vi "Monitor.vi"() -> ()   [LabVIEW 2017]
uses:
  Run_vi2.xctl
  <vilib>/Utility/miscctls.llb/LVPointTypeDef.ctl
  Global_comSerie.vi
  <vilib>/Instr/_visa.llb/VISA Configure Serial Port (Instr).vi
  GlobalFag.vi
  <vilib>/addons/database/Connection.llb/DB Tools Open Connec (Path).vi
  Global_linker_path_logger.vi
  contador_logger_global.vi
  global_act_eje_aula.vi
  global_act_eje_edif.vi
  Global_linker_path_3.vi
  <vilib>/addons/database/_DB Variant To Data/Database Variant To Data.xnode
  <vilib>/addons/database/NI_Database_API.lvlib
panel:
  in  "Periodo (s)":dbl=20.0 caption="Time Target (s)"
  out "Numeric":i32
  in  "Run_vi2":dbl(xcontrol)
  out "+/-_2":bool
  out "bit_edo_+/-_2":bool
  out "bit_edo_+/-":bool
  out "+/-":bool
  out "A_fin":u8
  out "A_ini":u8
  out "rango_TRUE":bool
  out "range":u8
  out "servicio_hex 2":string
  out "Edificio_ 2":string
  out "Hora_Inicio as string 2":string
  out "Hora_Inicio_as Time stamp 2":timestamp format="%<%X>T"
  out "Tarea Aula_ok":bool
  out "Aula":string
  out "ID a ejecutar":string
  out "hora_hoy as string 2":string
  out "Table Control_aulas":string[][](table) caption="Tarea por Aula"
  out "size_aulas":i32[](array[numeric])
  in  "Programar Tareas2":bool
  in  "Home Button":bool
  out "ID a ejecutar":string
  out "servicio_hex":string
  out "Edificio_":string
  out "Hora_Inicio as string":string
  out "Hora_Inicio_as Time stamp 1":timestamp format="%<%X>T"
  out "tarea_edif_ok":bool
  out "hora_hoy as string":string
  out "Table Control":string[][](table) caption="Tareas por Edificio"
  out "size(s)":i32[](array[numeric])
  in  "Ejecutor de Tareas":bool
  in  "Programar Tareas":bool
  out "inc_1":bool
  out "inc_2":bool
  out "inc_3":bool
  out "inc_4":bool
  out "inc_5":bool
  out "inc_6":bool
  out "inc_7":bool
  out "inc_8":bool
  out "inc_9":bool
  out "inc_10":bool
  out "inc_11":bool
  out "inc_12":bool
  out "inc_16":bool
  out "inc_15":bool
  out "inc_14":bool
  out "inc_13":bool
  in  "Puerto Serial":refnum<visa-resource-name>="COM1"
  out "A_16":bool[](array[boolean])
  out "A_15":bool[](array[boolean])
  out "A_14":bool[](array[boolean])
  out "A_13":bool[](array[boolean])
  out "A_12":bool[](array[boolean])
  out "A_11":bool[](array[boolean])
  out "A_10":bool[](array[boolean])
  out "A_9":bool[](array[boolean])
  out "A_8":bool[](array[boolean])
  out "A_7":bool[](array[boolean])
  out "A_6":bool[](array[boolean])
  out "A_5":bool[](array[boolean])
  out "A_4":bool[](array[boolean])
  out "A_3":bool[](array[boolean])
  out "A_2":bool[](array[boolean])
  out "A_1":bool[](array[boolean])
  in  "Stop Button":bool
  in  "Manual Aula / Edificio":bool
  # "Edificio A"
  # "Ejecutor de Tareas"
  # "a"
  # "b"
  # "c"
  # "d"
  # "e"
  # "Aula"
  # "1"
  # "a.- Luz\nb.- Aire\nc.- Proyector\nd.- Agua\ne.- Acceso"
  # "2"
  # "3"
  # "4"
  # "5"
  # "Servicios:"
  # "6"
  # "a  Luz"
  # "7"
  # "b  Aire"
  # "8"
  # "c  Proyector"
  # "d  Agua"
  # "9"
  # "e  Acceso"
  # "10"
  # "11"
  # "12"
  # "13"
  # "14"
  # "15"
  # "16"
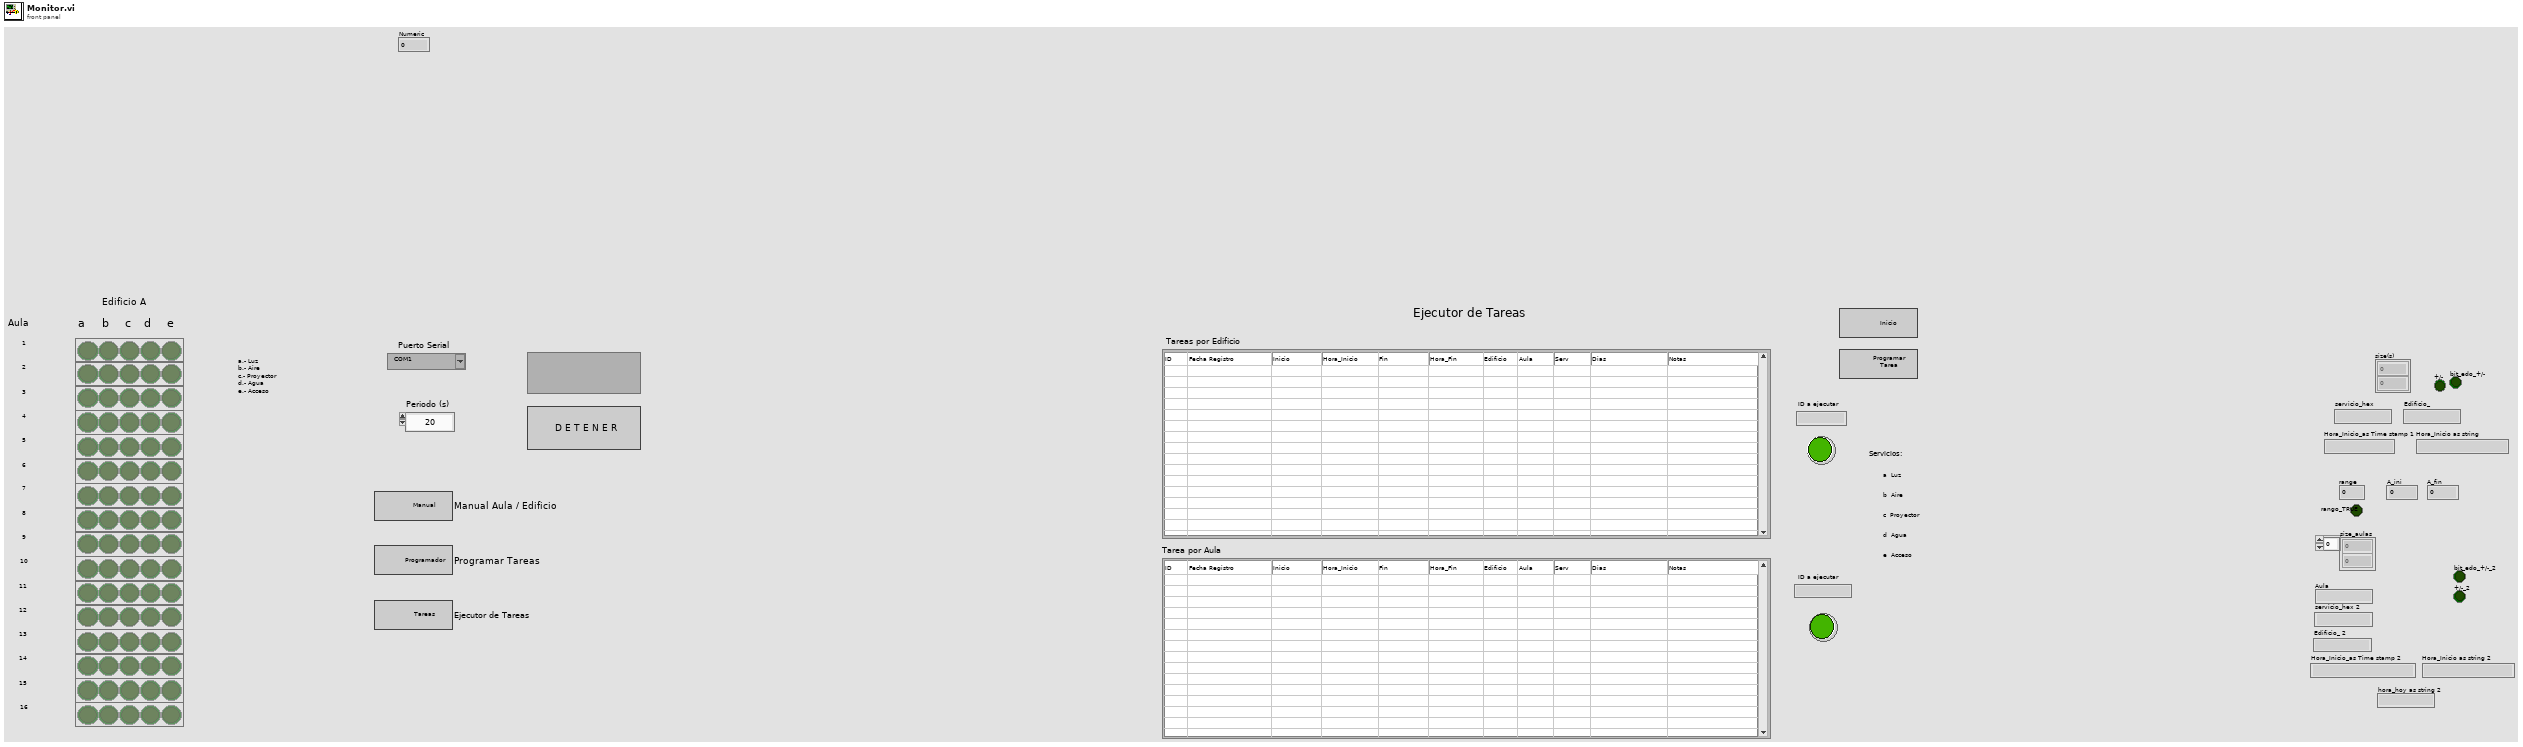
[diagram p1: front panel]
types:
  T1 = enum16{"open", "replace", "create", "open or create", "replace or create", "replace or create with confirmation"}
  T2 = typedef "LVPointTypeDef.ctl" = cluster{"Horizontal":i16, "Vertical":i16}
  T3 = typedef "NI_Database_API.lvlib/Conn ObjectReference.ctl" = refnum<k1>
  T4 = cluster{u64, string, "read buffer":string, u8, "serv":string}
  T5 = enum32{"Invalid", "Standard", "Closed", "Hidden", "Minimized", "Maximized"}
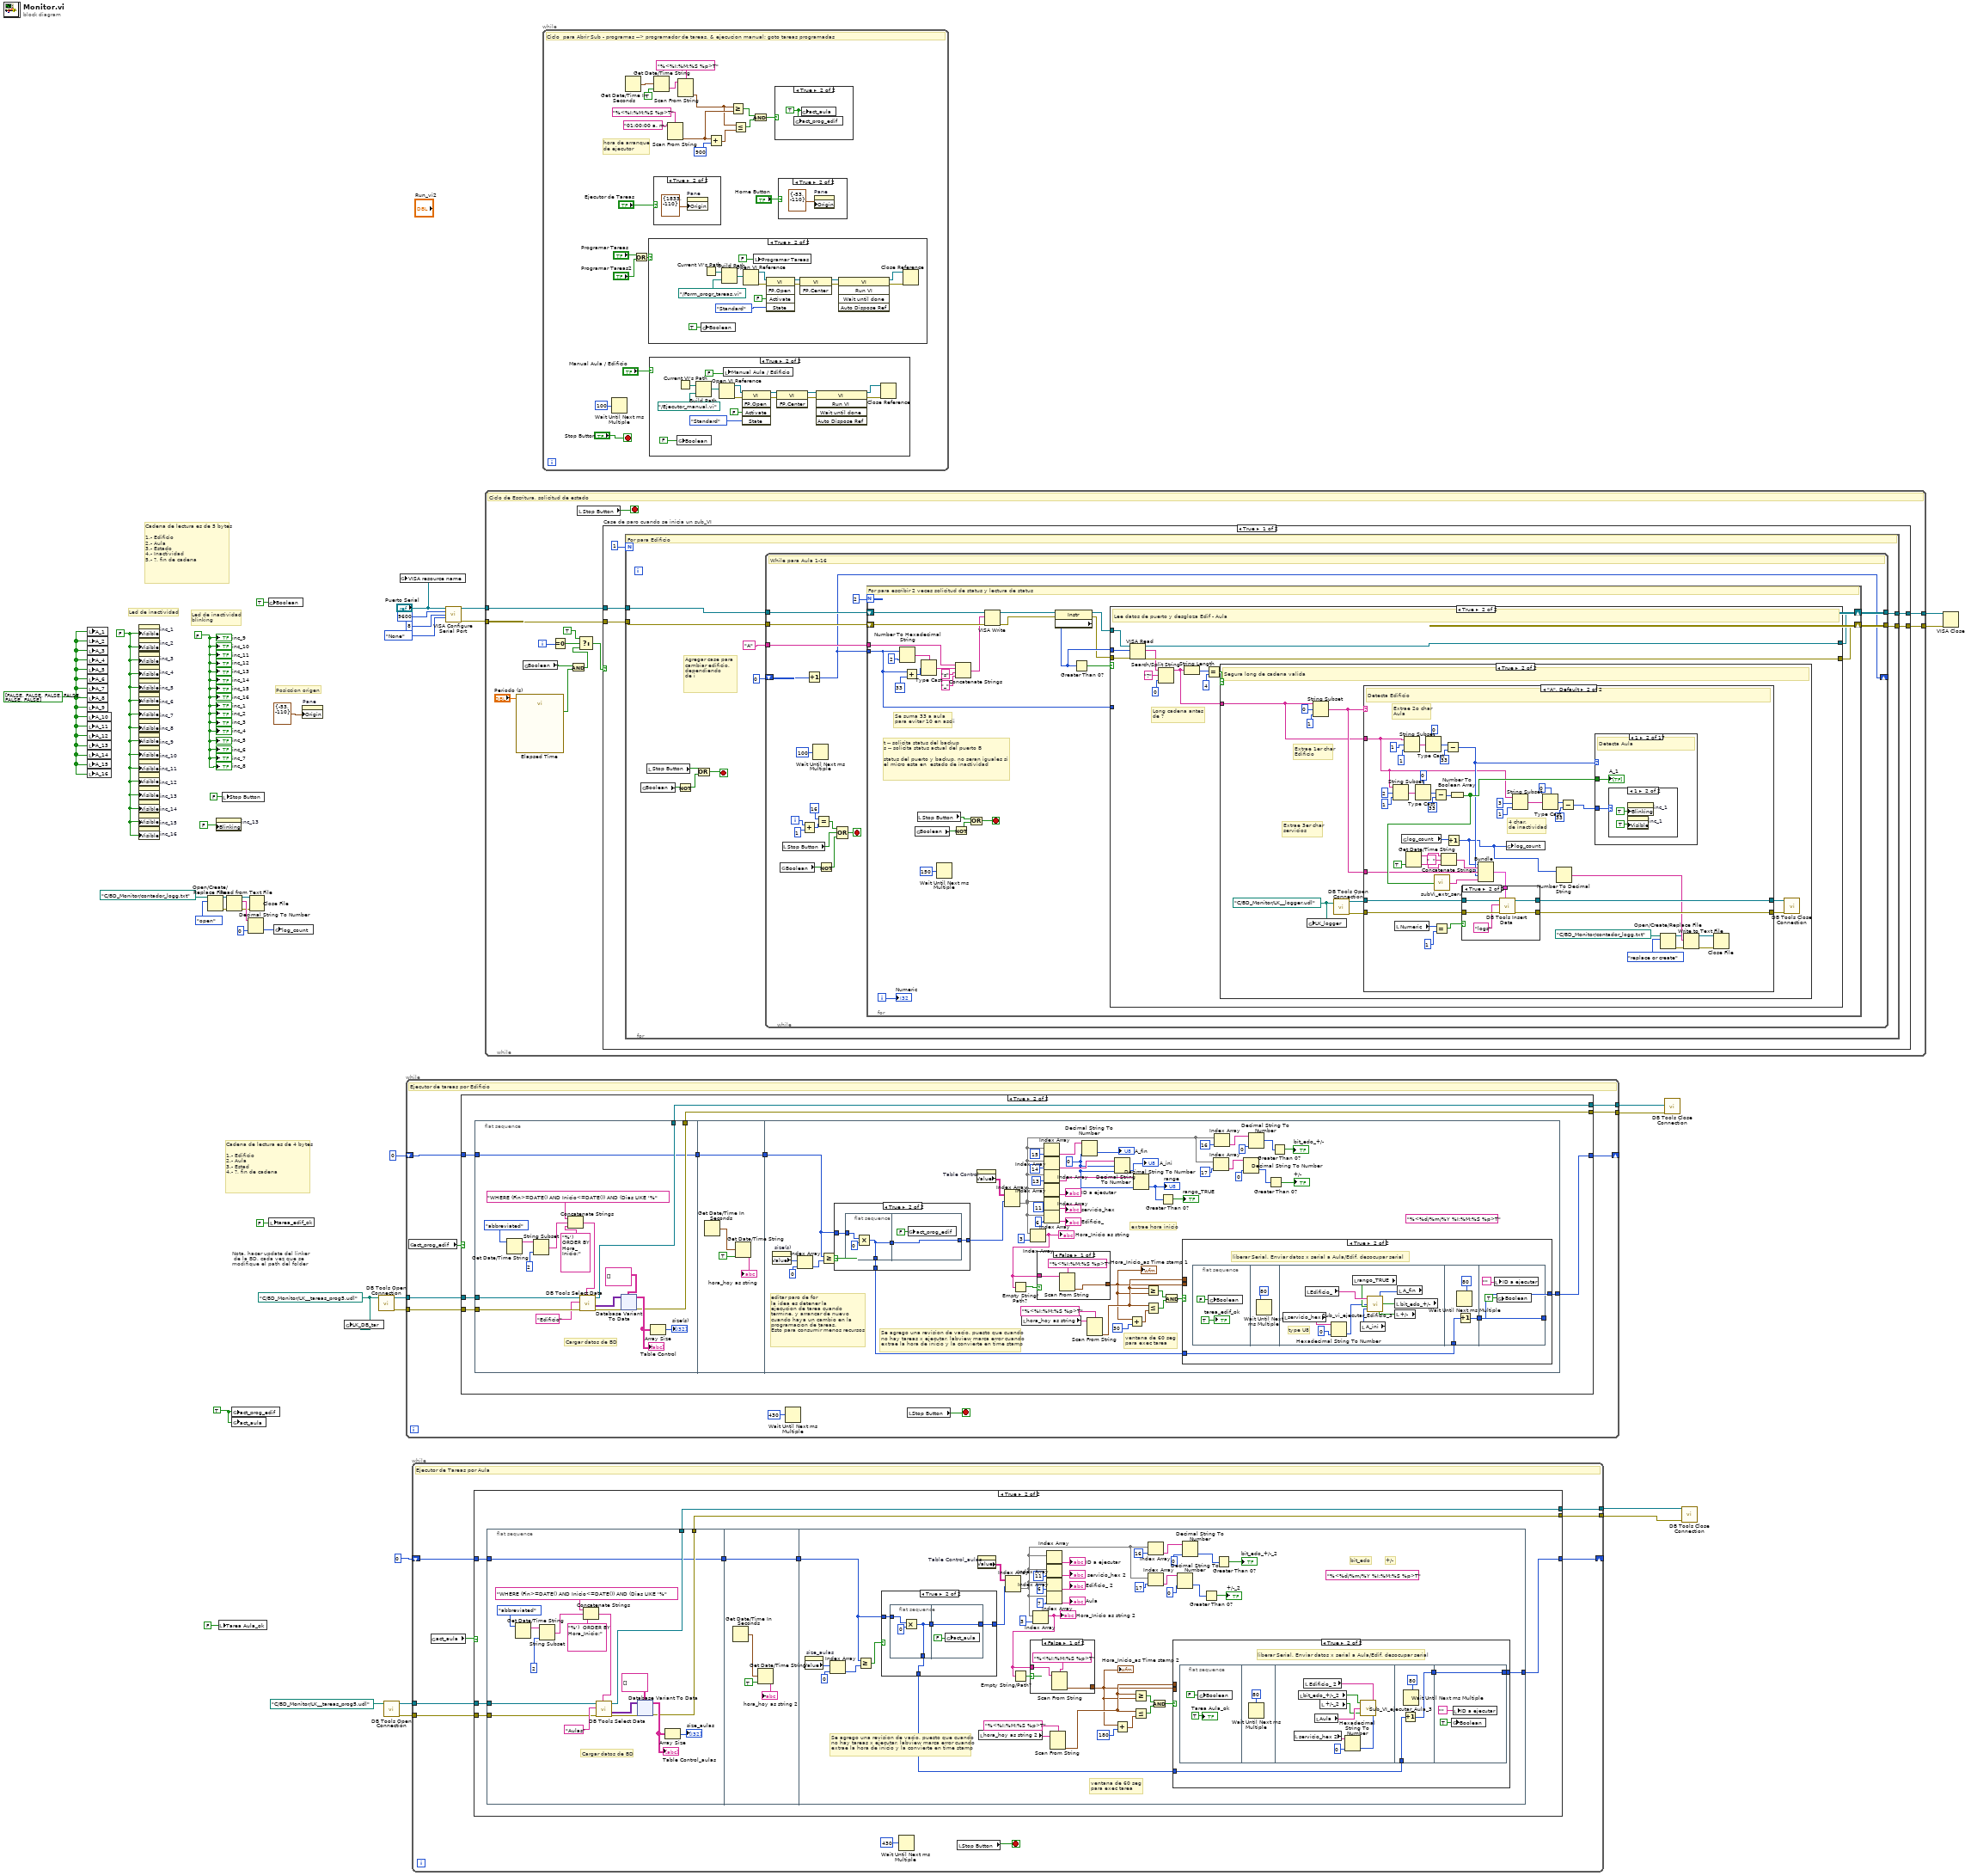
[diagram p0: block diagram]
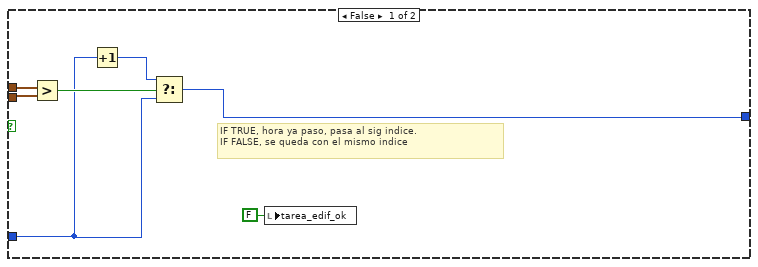
[diagram p4: hidden frame]
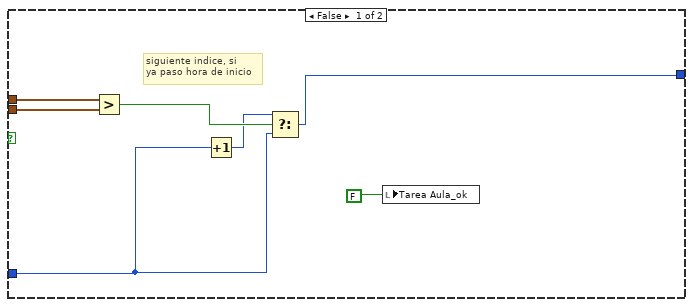
[diagram p8: hidden frame]
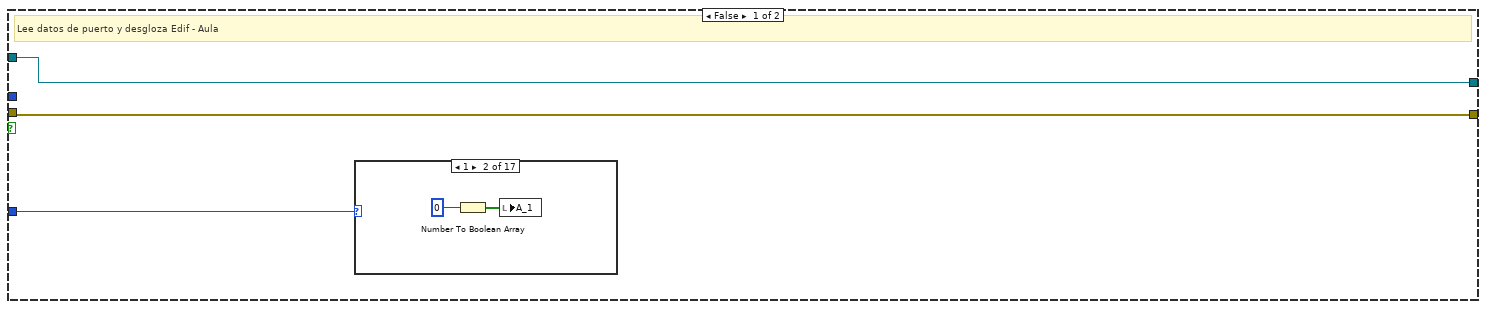
[diagram p15: hidden frame]
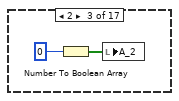
[diagram p17: hidden frame]
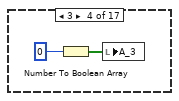
[diagram p18: hidden frame]
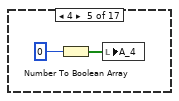
[diagram p19: hidden frame]
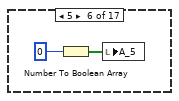
[diagram p20: hidden frame]
diagram:
  w2 = path "C:/BD_Monitor/LK__tareas_prog5.udl" ("path")
  w13 = TRUE ("act_prog_edif")
  w28 = FALSE ("Visible")
  w30 = FALSE ("Visible")
  w38 = bool[] [FALSE, FALSE, FALSE, FALSE, FALSE, FALSE] ("Edif A")
  # "Nota, hacer update del linker\n de la BD, cada vez que se \nmodifique el path del folder"
  # "Cadena de lectura es de 4 bytes\n\n1.- Edificio\n2.- Aula\n3.- Estad\n4.- ?, fin de cadena"
  # "Posiccion origen"
  # "Led de inactividad\nblinking"
  # "Led de inactividad"
  # "Cadena de lectura es de 5 bytes\n\n1.- Edificio\n2.- Aula\n3.- Estado\n4.- Inactividad\n5.- ?, fin de cadena"
  n1 = local write "A_1"(w38) -> ()
  n2 = local write "A_2"(w38) -> ()
  n3 = local write "A_3"(w38) -> ()
  n4 = local write "A_4"(w38) -> ()
  n5 = local write "A_5"(w38) -> ()
  n6 = local write "A_6"(w38) -> ()
  n7 = local write "A_7"(w38) -> ()
  n8 = local write "A_8"(w38) -> ()
  n9 = local write "A_9"(w38) -> ()
  n10 = local write "A_10"(w38) -> ()
  n11 = local write "A_11"(w38) -> ()
  n12 = local write "A_12"(w38) -> ()
  n13 = local write "A_13"(w38) -> ()
  n14 = local write "A_14"(w38) -> ()
  n15 = local write "A_15"(w38) -> ()
  n16 = local write "A_16"(w38) -> ()
  n17 = property on="inc_1" class="Bool (strict)"("Visible"=w30) -> ()  [unwired: 2 in, 2 out]
  n18 = property on="inc_2" class="Bool (strict)"("Visible"=w30) -> ()  [unwired: 2 in, 2 out]
  n19 = property on="inc_3" class="Bool (strict)"("Visible"=w30) -> ()  [unwired: 2 in, 2 out]
  n20 = property on="inc_4" class="Bool (strict)"("Visible"=w30) -> ()  [unwired: 2 in, 2 out]
  n21 = property on="inc_5" class="Bool (strict)"("Visible"=w30) -> ()  [unwired: 2 in, 2 out]
  n22 = property on="inc_6" class="Bool (strict)"("Visible"=w30) -> ()  [unwired: 2 in, 2 out]
  n23 = property on="inc_7" class="Bool (strict)"("Visible"=w30) -> ()  [unwired: 2 in, 2 out]
  n24 = property on="inc_8" class="Bool (strict)"("Visible"=w30) -> ()  [unwired: 2 in, 2 out]
  n25 = property on="inc_9" class="Bool (strict)"("Visible"=w30) -> ()  [unwired: 2 in, 2 out]
  n26 = property on="inc_10" class="Bool (strict)"("Visible"=w30) -> ()  [unwired: 2 in, 2 out]
  n27 = property on="inc_11" class="Bool (strict)"("Visible"=w30) -> ()  [unwired: 2 in, 2 out]
  n28 = property on="inc_12" class="Bool (strict)"("Visible"=w30) -> ()  [unwired: 2 in, 2 out]
  n29 = property on="inc_13" class="Bool (strict)"("Visible"=w30) -> ()  [unwired: 2 in, 2 out]
  n30 = property on="inc_14" class="Bool (strict)"("Visible"=w30) -> ()  [unwired: 2 in, 2 out]
  n31 = property on="inc_15" class="Bool (strict)"("Visible"=w30) -> ()  [unwired: 2 in, 2 out]
  n32 = property on="inc_16" class="Bool (strict)"("Visible"=w30) -> ()  [unwired: 2 in, 2 out]
  n33 = Open/Create/Replace File(file path (use dialog)=path "C:/BD_Monitor/contador_logg.txt" ("path"), operation (0:open)=T1."open") -> (refnum out=w10:refnum<file>, error out=w11:errorcluster)  [unwired: 4 in, 1 out]
  n34 = property on="inc_13" class="Bool (strict)"("Blinking"=FALSE) -> ()  [unwired: 2 in, 2 out]
  n35 = local write "Tarea Aula_ok"(FALSE ("Loading")) -> ()
  n36 = local write "Stop Button"(FALSE ("Stop Button")) -> ()
  n37 = Read from Text File(file (use dialog)=w10, error in=w11) -> (refnum out=w9:refnum<file>, text=w12:string, error out=w8:errorcluster)  [unwired: 2 in, 1 out]
  n38 = global write "global_act_eje_edif.vi" "act_prog_edif"(w13) -> ()
  n39 = global write "global_act_eje_aula.vi" "act_aula"(w13) -> ()
  n40 = Decimal String To Number(string=w12, default (0L)=u64 0 ("default (0 I32)")) -> (number=w6:u64)  [unwired: 1 in, 1 out]
  n41 = Close File(refnum=w9, error in=w8) -> ()  [unwired: 2 out]
  n42 = global write "GlobalFag.vi" "Boolean"(TRUE ("Boolean")) -> ()
  n43 = local write "tarea_edif_ok"(FALSE ("Loading")) -> ()
  n44 = global write "contador_logger_global.vi" "log_count"(w6) -> ()
  n45 = property on="Pane" class="Pane"("Origin"=T2 {"Horizontal"=-53, "Vertical"=-110}) -> ()  [unwired: 2 in, 2 out]
  n46 = global write "Global_linker_path_3.vi" "LK_DB_tar"(w2) -> ()
  n47 = call-poly <vilib>:"DB Tools Open Connection.vi"("connection information"=w2) -> ("error out"=w18:errorcluster, "connection reference"=w19:T3)  [unwired: 7 in]
  n48 = call-poly <vilib>:"DB Tools Open Connection.vi"("connection information"=path "C:/BD_Monitor/LK__tareas_prog5.udl" ("path")) -> ("error out"=w24:errorcluster, "connection reference"=w23:T3)  [unwired: 7 in]
  n49 = global write "Global_comSerie.vi" "VISA resource name"("Puerto Serial") -> ()
  n50 = while {
    shift-right: [w43] -> _
    shift-left: 0 ("index") -> [w44]
    tunnel: w18 -> [w48]
    tunnel: w19 -> [w47]
    tunnel: [w46] -> w15
    tunnel: [w45] -> w14
    stop <- w41 stop-if-true
    # "Ejecutor de tareas por Edificio"
    n51 = global read "global_act_eje_edif.vi" "act_prog_edif"() -> (w42:bool)
    n52 = case shown="True" w42 {
      tunnel: w48 -> [w50 w57]
      tunnel: w47 -> [w51 w56]
      tunnel: [w50 w55] -> w46
      tunnel: [w51 w54] -> w45
      tunnel: w44 -> [w49 w53]
      tunnel: [w49 w52] -> w43
      frame False {
      }
      frame True {
        n53 = flat-sequence {
          tunnel: w53 -> [w60]
          tunnel: [w60] -> w59
          tunnel: w57 -> [w65]
          tunnel: w56 -> [w63]
          tunnel: [w62] -> w54
          tunnel: [w61] -> w55
          tunnel: [w125] -> w58
          tunnel: w59 -> [w125]
          tunnel: w58 -> [w154]
          tunnel: [w151] -> w52
          frame #0 {
            # "Cargar datos de BD"
            n54 = Get Date/Time String(date format (0)=enum16{"short", "long", "abbreviated"}."abbreviated") -> (date string=w71:string)  [unwired: 2 in, 1 out]
            n55 = String Subset(string=w71, length (rest)=2 ("length (rest)")) -> (substring=w72:string)  [unwired: 1 in]
            n56 = Concatenate Strings("WHERE (Fin>=DATE() AND Inicio<=DATE()) AND (Dias LIKE '%", w72, "%')  ORDER BY Hora_Inicio;") -> (w75:string)
            n57 = call <vilib>:"DB Tools Select Data.vi"("condition"=w75, "error in (no error)"=w65, "table"="Edificio", "connection reference"=w63) -> ("error out"=w73:errorcluster, "data"=w74:variant[][], "connection reference out"=w62:T3)  [unwired: 2 in]
            n58 = xnode "Database Variant To Data"("database variant"=w74, "error in (no error)"=w73, "type"=string[][] []) -> ("data"=w76:string[][], "error out"=w61:errorcluster)
            "Table Control" <- w76
            n59 = Array Size(array=w76) -> (size(s)=→"size(s)":i32[])
          }
          frame #1 {
            n60 = Get Date/Time In Seconds() -> (seconds since 1Jan1904=w123:timestamp)
            n61 = Get Date/Time String(seconds (now)=w123, want seconds? (F)=TRUE) -> (time string=→"hora_hoy as string":string)  [unwired: 1 in, 1 out]
          }
          frame #2 {
            w144 = u8 0
            (unwired) "%<%d/%m/%Y %I:%M:%S %p>T" ("format string")
            # "Se agrego una revision de vacio, puesto que cuando\nno hay tareas x ejecutar, labview marca error cuando \nextrae la hora de inicio y la convierte en time stamp"
            # "editar paro de for\nla idea es detener la\nejecucion de tarea cuando\ntermine, y arrancar de nuevo\ncuando haya un cambio en la\nprogramacion de tareas.\nEsto para consumir menos recursos"
            # "ventana de 60 seg para exec tarea"
            # "extrae hora inicio"
            n62 = property on="size(s)" class="Arr (strict)"() -> ("Value"=w169:i32[])  [unwired: 2 in, 2 out]
            n63 = Index Array(array=w169, index=0) -> (element=w170:i32)
            n64 = Greater Or Equal?(x=w154, y=w170) -> (x >= y?=w161:bool)
            n65 = case shown="True" w161 {
              tunnel: [w205 w206] -> w171
              tunnel: [w205 w208] -> w152
              tunnel: w154 -> [w205 w209]
              frame False {
              }
              frame True {
                n66 = flat-sequence {
                  tunnel: [w210] -> w208
                  tunnel: w209 -> [w212]
                  tunnel: [w210] -> w207
                  tunnel: w207 -> [w213]
                  tunnel: [w213] -> w206
                  frame #0 {
                    n67 = Multiply(x=w212, y=0 ("index")) -> (x*y=w210:i32)
                  }
                  frame #1 {
                    n68 = global write "global_act_eje_edif.vi" "act_prog_edif"(FALSE ("Boolean")) -> ()
                  }
                }
              }
            }
            n69 = property on="Table Control" class="Tbl (strict)"() -> ("Value"=w167:string[][])  [unwired: 2 in, 2 out]
            n70 = Index Array(array=w167, index (row)=w171) -> (element=w133:string[])  [unwired: 1 in]
            n71 = local read "hora_hoy as string"() -> (w173:string)
            n72 = Index Array(array=w133, index=3 ("index (row)")) -> (element=w126:string)
            "Hora_Inicio as string" <- w126
            n73 = Empty String/Path?(string/path=w126) -> (empty?=w128:bool)
            n74 = case shown="False" w128 {
              tunnel: [w175 _] -> w127
              tunnel: w126 -> [w174 _]
              frame False {
                n75 = Scan From String(format string="%<%I:%M:%S %p>T", input string=w174) -> (output 1=w175:timestamp)  [unwired: 3 in, 3 out]
              }
              frame True {
              }
            }
            "Hora_Inicio_as Time stamp 1" <- w127
            n76 = Index Array(array=w133, index=15 ("index (row)")) -> (element=w145:string)
            n77 = Index Array(array=w133, index=14 ("index (row)")) -> (element=w146:string)
            n78 = Index Array(array=w133, index=13 ("index (row)")) -> (element=w147:string)
            n79 = Index Array(array=w133) -> (element=→"ID a ejecutar":string)  [unwired: 1 in]
            n80 = Index Array(array=w133, index=11 ("index (row)")) -> (element=→"servicio_hex":string)
            n81 = Index Array(array=w133, index=6 ("index (row)")) -> (element=→"Edificio_":string)
            n82 = Decimal String To Number(string=w145, default (0L)=w144) -> (number=→"A_fin":u8)  [unwired: 1 in, 1 out]
            n83 = Scan From String(format string="%<%I:%M:%S %p>T", input string=w173) -> (output 1=w155:timestamp)  [unwired: 3 in, 3 out]
            n84 = Decimal String To Number(string=w146, offset=w144, default (0L)=w144) -> (number=→"A_ini":u8)  [unwired: 1 out]
            n85 = Add(x=w127, y=30) -> (x+y=w160:timestamp)
            n86 = Decimal String To Number(string=w147, default (0L)=w144) -> (number=w143:u8)  [unwired: 1 in, 1 out]
            "range" <- w143
            n87 = Greater Or Equal?(x=w155, y=w127) -> (x >= y?=w156:bool)
            n88 = Less Or Equal?(x=w155, y=w160) -> (x <= y?=w157:bool)
            n89 = Greater Than 0?(x=w143) -> (x > 0?=→"rango_TRUE":bool)
            n90 = And(x=w156, y=w157) -> (x .and. y?=w158:bool)
            n91 = case shown="True" w158 {
              tunnel: w152 -> [w178 w186]
              tunnel: w155 -> [w180 _]
              tunnel: w127 -> [w179 _]
              tunnel: [w177 w184] -> w151
              frame False {
                # "IF TRUE, hora ya paso, pasa al sig indice.\nIF FALSE, se queda con el mismo indice"
                n92 = Greater?(x=w180, y=w179) -> (0:w182:bool)
                n93 = Increment(x=w178) -> (x+1=w181:i32)
                n94 = Select(t=w181, s=w182, f=w178) -> (s? t:f=w177:i32)
                n95 = local write "tarea_edif_ok"(FALSE) -> ()
              }
              frame True {
                # "liberar Serial, Enviar datos x serial a Aula/Edif, desocupar serial"
                n96 = flat-sequence {
                  tunnel: w186 -> [w200]
                  tunnel: [w201] -> w185
                  tunnel: [w204] -> w184
                  tunnel: w185 -> [w204]
                  frame #0 {
                    n97 = global write "GlobalFag.vi" "Boolean"(FALSE ("Boolean")) -> ()
                    "tarea_edif_ok" <- TRUE
                  }
                  frame #1 {
                    n98 = Wait Until Next ms Multiple(millisecond multiple=u32 80) -> ()  [unwired: 1 out]
                  }
                  frame #2 {
                    # "type U8"
                    n99 = local read "servicio_hex"() -> (w198:string)
                    n100 = local read "Edificio_"() -> (w194:string)
                    n101 = Hexadecimal String To Number(string=w198, default (0uL)=u8 0 ("index")) -> (number=w191:u8)  [unwired: 1 in, 1 out]
                    n102 = local read "rango_TRUE"() -> (w193:bool)
                    n103 = local read "A_ini"() -> (w190:u8)
                    n104 = local read "bit_edo_+/-"() -> (w196:bool)
                    n105 = local read "+/-"() -> (w195:bool)
                    n106 = local read "A_fin"() -> (w192:u8)
                    n107 = call "Sub_vi_ejecutar_Edificio_3.vi"("Edificio_string"=w194, "Serv_Numeric"=w191, "De"=w190, "Hasta"=w192, "edo_actual_aula"=w196, "rango"=w193, "+                 -"=w195) -> ()
                  }
                  frame #3 {
                    n108 = Wait Until Next ms Multiple(millisecond multiple=u32 80) -> ()  [unwired: 1 out]
                    n109 = Increment(x=w200) -> (x+1=w201:i32)
                  }
                  frame #4 {
                    n110 = local write "ID a ejecutar"("") -> ()
                    n111 = global write "GlobalFag.vi" "Boolean"(TRUE ("Boolean")) -> ()
                  }
                }
              }
            }
            n112 = Index Array(array=w133, index=17 ("index (row)")) -> (element=w138:string)
            n113 = Index Array(array=w133, index=16 ("index (row)")) -> (element=w136:string)
            n114 = Decimal String To Number(string=w138, default (0L)=u8 0) -> (number=w132:u8)  [unwired: 1 in, 1 out]
            n115 = Decimal String To Number(string=w136, default (0L)=u8 0) -> (number=w130:u8)  [unwired: 1 in, 1 out]
            n116 = Greater Than 0?(x=w132) -> (x > 0?=→"+/-":bool)
            n117 = Greater Than 0?(x=w130) -> (x > 0?=→"bit_edo_+/-":bool)
          }
        }
      }
    }
    n118 = Wait Until Next ms Multiple(millisecond multiple=u32 430) -> ()  [unwired: 1 out]
    n119 = local read "Stop Button"() -> (w41:bool)
  }
  n120 = while {
    tunnel: w24 -> [w223]
    tunnel: w23 -> [w222]
    tunnel: [w220] -> w22
    tunnel: [w221] -> w21
    shift-right: [w217] -> _
    shift-left: 0 ("index") -> [w219]
    stop <- w216 stop-if-true
    # "Ejecutor de Tareas por Aula"
    n121 = global read "global_act_eje_aula.vi" "act_aula"() -> (w215:bool)
    n122 = case shown="True" w215 {
      tunnel: w223 -> [w225 w232]
      tunnel: w222 -> [w224 w231]
      tunnel: [w225 w230] -> w221
      tunnel: [w224 w229] -> w220
      tunnel: w219 -> [w226 w228]
      tunnel: [w226 w227] -> w217
      frame False {
      }
      frame True {
        n123 = flat-sequence {
          tunnel: w232 -> [w239]
          tunnel: w231 -> [w238]
          tunnel: [w237] -> w230
          tunnel: [w236] -> w229
          tunnel: [w235] -> w234
          tunnel: w228 -> [w235]
          tunnel: [w297] -> w233
          tunnel: w234 -> [w297]
          tunnel: w233 -> [w315]
          tunnel: [w314] -> w227
          frame #0 {
            # "Cargar datos de BD"
            n124 = Get Date/Time String(date format (0)=enum16{"short", "long", "abbreviated"}."abbreviated") -> (date string=w251:string)  [unwired: 2 in, 1 out]
            n125 = String Subset(string=w251, length (rest)=2 ("length (rest)")) -> (substring=w249:string)  [unwired: 1 in]
            n126 = Concatenate Strings("WHERE (Fin>=DATE() AND Inicio<=DATE()) AND (Dias LIKE '%", w249, "%')  ORDER BY Hora_Inicio;") -> (w243:string)
            n127 = call <vilib>:"DB Tools Select Data.vi"("condition"=w243, "error in (no error)"=w239, "table"="Aulas", "connection reference"=w238) -> ("error out"=w247:errorcluster, "data"=w246:variant[][], "connection reference out"=w236:T3)  [unwired: 2 in]
            n128 = xnode "Database Variant To Data"("database variant"=w246, "error in (no error)"=w247, "type"=string[][] []) -> ("data"=w241:string[][], "error out"=w237:errorcluster)
            "Table Control_aulas" <- w241
            n129 = Array Size(array=w241) -> (size(s)=→"size_aulas":i32[])
          }
          frame #1 {
            n130 = Get Date/Time In Seconds() -> (seconds since 1Jan1904=w300:timestamp)
            n131 = Get Date/Time String(seconds (now)=w300, want seconds? (F)=TRUE) -> (time string=→"hora_hoy as string 2":string)  [unwired: 1 in, 1 out]
          }
          frame #2 {
            (unwired) "%<%d/%m/%Y %I:%M:%S %p>T" ("format string")
            # "Se agrego una revision de vacio, puesto que cuando\nno hay tareas x ejecutar, labview marca error cuando \nextrae la hora de inicio y la convierte en time stamp"
            # "+/-"
            # "bit_edo"
            # "ventana de 60 seg para exec tarea"
            n132 = property on="size_aulas" class="Arr (strict)"() -> ("Value"=w335:i32[])  [unwired: 2 in, 2 out]
            n133 = Index Array(array=w335, index=0) -> (element=w336:i32)
            n134 = Greater Or Equal?(x=w315, y=w336) -> (x >= y?=w328:bool)
            n135 = case shown="True" w328 {
              tunnel: [w369 w370] -> w337
              tunnel: [w369 w373] -> w327
              tunnel: w315 -> [w369 w372]
              frame False {
              }
              frame True {
                n136 = flat-sequence {
                  tunnel: [w374] -> w373
                  tunnel: w372 -> [w376]
                  tunnel: [w374] -> w371
                  tunnel: w371 -> [w378]
                  tunnel: [w378] -> w370
                  frame #0 {
                    n137 = Multiply(x=w376, y=0 ("index")) -> (x*y=w374:i32)
                  }
                  frame #1 {
                    n138 = global write "global_act_eje_aula.vi" "act_aula"(FALSE ("act_aula")) -> ()
                  }
                }
              }
            }
            n139 = property on="Table Control_aulas" class="Tbl (strict)"() -> ("Value"=w333:string[][])  [unwired: 2 in, 2 out]
            n140 = local read "hora_hoy as string 2"() -> (w339:string)
            n141 = Index Array(array=w333, index (row)=w337) -> (element=w313:string[])  [unwired: 1 in]
            n142 = Index Array(array=w313, index=3 ("index (row)")) -> (element=w301:string)
            "Hora_Inicio as string 2" <- w301
            n143 = Empty String/Path?(string/path=w301) -> (empty?=w302:bool)
            n144 = case shown="False" w302 {
              tunnel: [w342 _] -> w320
              tunnel: w301 -> [w340 _]
              frame False {
                n145 = Scan From String(format string="%<%I:%M:%S %p>T", input string=w340) -> (output 1=w342:timestamp)  [unwired: 3 in, 3 out]
              }
              frame True {
              }
            }
            "Hora_Inicio_as Time stamp 2" <- w320
            n146 = Index Array(array=w313) -> (element=→"ID a ejecutar":string)  [unwired: 1 in]
            n147 = Index Array(array=w313, index=11 ("index (row)")) -> (element=→"servicio_hex 2":string)
            n148 = Index Array(array=w313, index=6 ("index (row)")) -> (element=→"Edificio_ 2":string)
            n149 = Index Array(array=w313, index=7 ("index (row)")) -> (element=→"Aula":string)
            n150 = Scan From String(format string="%<%I:%M:%S %p>T", input string=w339) -> (output 1=w321:timestamp)  [unwired: 3 in, 3 out]
            n151 = Add(x=w320, y=180) -> (x+y=w326:timestamp)
            n152 = Greater Or Equal?(x=w321, y=w320) -> (x >= y?=w322:bool)
            n153 = Less Or Equal?(x=w321, y=w326) -> (x <= y?=w323:bool)
            n154 = Index Array(array=w313, index=16 ("index (row)")) -> (element=w310:string)
            n155 = Index Array(array=w313, index=17 ("index (row)")) -> (element=w308:string)
            n156 = And(x=w322, y=w323) -> (x .and. y?=w324:bool)
            n157 = case shown="True" w324 {
              tunnel: w327 -> [w344 w350]
              tunnel: w321 -> [w346 _]
              tunnel: w320 -> [w345 _]
              tunnel: [w343 w352] -> w314
              frame False {
                # "siguiente indice, si \nya paso hora de inicio"
                n158 = Greater?(x=w346, y=w345) -> (0:w348:bool)
                n159 = Increment(x=w344) -> (x+1=w347:i32)
                n160 = Select(t=w347, s=w348, f=w344) -> (s? t:f=w343:i32)
                n161 = local write "Tarea Aula_ok"(FALSE) -> ()
              }
              frame True {
                # "liberar Serial, Enviar datos x serial a Aula/Edif, desocupar serial"
                n162 = flat-sequence {
                  tunnel: [w365] -> w351
                  tunnel: w350 -> [w363]
                  tunnel: [w368] -> w352
                  tunnel: w351 -> [w368]
                  frame #0 {
                    n163 = global write "GlobalFag.vi" "Boolean"(FALSE ("Boolean")) -> ()
                    "Tarea Aula_ok" <- TRUE
                  }
                  frame #1 {
                    n164 = Wait Until Next ms Multiple(millisecond multiple=u32 80) -> ()  [unwired: 1 out]
                  }
                  frame #2 {
                    n165 = local read "servicio_hex 2"() -> (w362:string)
                    n166 = local read "bit_edo_+/-_2"() -> (w357:bool)
                    n167 = local read "Edificio_ 2"() -> (w360:string)
                    n168 = local read "Aula"() -> (w359:string)
                    n169 = local read "+/-_2"() -> (w356:bool)
                    n170 = Hexadecimal String To Number(string=w362, default (0uL)=u8 0 ("index")) -> (number=w358:u8)  [unwired: 1 in, 1 out]
                    n171 = call "Sub_VI_ejecutar_Aula_3.vi"("Serrvicio"=w358, "Edif_string_aula"=w360, "+                 -"=w356, "Aula"=w359, "edo_actual_aula"=w357) -> ()
                  }
                  frame #3 {
                    n172 = Increment(x=w363) -> (x+1=w365:i32)
                    n173 = Wait Until Next ms Multiple(millisecond multiple=u32 80) -> ()  [unwired: 1 out]
                  }
                  frame #4 {
                    n174 = global write "GlobalFag.vi" "Boolean"(TRUE ("Boolean")) -> ()
                    n175 = local write "ID a ejecutar"("") -> ()
                  }
                }
              }
            }
            n176 = Decimal String To Number(string=w308, default (0L)=u8 0) -> (number=w304:u8)  [unwired: 1 in, 1 out]
            n177 = Decimal String To Number(string=w310, default (0L)=u8 0) -> (number=w306:u8)  [unwired: 1 in, 1 out]
            n178 = Greater Than 0?(x=w304) -> (x > 0?=→"+/-_2":bool)
            n179 = Greater Than 0?(x=w306) -> (x > 0?=→"bit_edo_+/-_2":bool)
          }
        }
      }
    }
    n180 = Wait Until Next ms Multiple(millisecond multiple=u32 430) -> ()  [unwired: 1 out]
    n181 = local read "Stop Button"() -> (w216:bool)
  }
  n182 = call-poly "VISA Configure Serial Port"("VISA resource name"="Puerto Serial", "baud rate (9600)"=u32 9600, "data bits (8)"=u16 8, "parity (0:none)"=enum16{"None", "Odd", "Even", "Mark", "Space"}."None") -> ("VISA resource name out"=w36:refnum<visa-resource-name>, "error out"=w35:errorcluster)  [unwired: 10 in]
  n183 = while "Ciclo de Escritura" {
    tunnel: w36 -> [w391]
    tunnel: w35 -> [w390]
    tunnel: [w389] -> w39
    tunnel: [w388] -> w37
    i -> [w383]
    stop <- w387 stop-if-true
    # "Ciclo de Escritura, solicitud de estado"
    n184 = call "Elapsed Time"("Time Target (s)"="Periodo (s)") -> ("Time has Elapsed"=w384:bool)  [unwired: 11 in, 7 out]
    n185 = global read "GlobalFag.vi" "Boolean"() -> (w385:bool)
    n186 = Equal To 0?(x=w383) -> (x = 0?=w382:bool)
    n187 = And(x=w385, y=w384) -> (x .and. y?=w380:bool)
    n188 = local read "Stop Button"() -> (w387:bool)
    n189 = Select(t=TRUE, s=w382, f=w380) -> (s? t:f=w379:bool)
    n190 = case "Case de paro cuando se inicia un sub_VI" shown="True" w379 {
      tunnel: [w393 w660] -> w389
      tunnel: [w392 w661] -> w388
      tunnel: w391 -> [w396 w660]
      tunnel: w390 -> [w395 w661]
      frame True {
        n191 = for {
          N: 1 -> [_]
          tunnel: w396 -> [w406]
          tunnel: w395 -> [w405]
          tunnel: [w404] -> w393
          tunnel: [w403] -> w392
          stop <- w402 stop-if-true
          # "Agregar case para \ncambiar edificio, \ndependiendo\nde i"
          # "For para Edificio"
          n192 = global read "GlobalFag.vi" "Boolean"() -> (w398:bool)
          n193 = local read "Stop Button"() -> (w399:bool)
          n194 = Not(x=w398) -> (.not. x?=w397:bool)
          n195 = Compound Arithmetic op=OR(w399, w397) -> (w402:bool)
          n196 = while {
            tunnel: "A" -> [w424]
            tunnel: w406 -> [w423]
            tunnel: w405 -> [w422]
            tunnel: [w421] -> w404
            shift-right: [w419] -> _
            shift-left: u8 0 ("width (-)") -> [w420]
            tunnel: [w418] -> w403
            i -> [w413]
            stop <- w415 stop-if-true
            # "While para Aula 1-16"
            n197 = global read "GlobalFag.vi" "Boolean"() -> (w408:bool)
            n198 = local read "Stop Button"() -> (w414:bool)
            n199 = Add(x=w413, y=1) -> (x+y=w411:i32)
            n200 = Increment(x=w420) -> (x+1=w419:u8)
            n201 = Wait Until Next ms Multiple(millisecond multiple=u32 100) -> ()  [unwired: 1 out]
            n202 = Equal?(x=16, y=w411) -> (x = y?=w416:bool)
            n203 = Not(x=w408) -> (.not. x?=w407:bool)
            n204 = Compound Arithmetic op=OR(w416, w414, w407) -> (w415:bool)
            n205 = for {
              N: 2 -> [_]
              tunnel: w424 -> [w450]
              tunnel: w419 -> [w429]
              shift-right: [w433] -> w421
              shift-left: w423 -> [w444]
              shift-right: [w432] -> w418
              shift-left: w422 -> [w443]
              i -> [w427]
              stop <- w430 stop-if-true
              # "t -- solicita status del backup\ns -- solicita status actual del puerto B\n\nstatus del puerto y backup, no seran iguales si \nel micro esta en  estado de inactividad"
              # "Se suma 33 a aula\npara evitar 10 en ascii"
              # "For para escribir 2 veces solicitud de status y lectura de status"
              n206 = Number To Hexadecimal String(1:u8 2 ("width (-)"), 2:w429) -> (0:w447:string)
              n207 = Add(x=w429, y=u8 33 ("width (-)")) -> (x+y=w441:u8)
              n208 = global read "GlobalFag.vi" "Boolean"() -> (w426:bool)
              n209 = local read "Stop Button"() -> (w431:bool)
              n210 = Type Cast(type=w447, x=w441) -> (*(type *) &x=w449:string)
              n211 = Wait Until Next ms Multiple(millisecond multiple=u32 150) -> ()  [unwired: 1 out]
              n212 = Not(x=w426) -> (.not. x?=w425:bool)
              n213 = Concatenate Strings(w450, w449, "s" ("string"), "_" ("string")) -> (w440:string)
              n214 = Compound Arithmetic op=OR(w431, w425) -> (w430:bool)
              n215 = VISA Write(VISA resource name=w444, write buffer=w440, error in (no error)=w443) -> (VISA resource name out=w435:refnum<visa-resource-name>, error out=w434:errorcluster)  [unwired: 1 out]
              n216 = property class="Instr"(reference=w435, error in=w434) -> (reference out=w428:refnum<visa-resource-name>, error out=w437:errorcluster, "Serial Settings:Number of Bytes at Serial Port"=w438:u32)
              n217 = Greater Than 0?(x=w438) -> (x > 0?=w436:bool)
              n218 = case shown="True" w436 {
                tunnel: w437 -> [w453 w497]
                tunnel: w438 -> [_ w496]
                tunnel: [w451 w495] -> w433
                tunnel: [w453 w494] -> w432
                tunnel: w429 -> [w452 _]
                tunnel: w428 -> [w451 w486]
                frame False {
                  # "Lee datos de puerto y desgloza Edif - Aula"
                  n219 = case shown="1" w452 {
                    frame 0, Default {
                    }
                    frame 1 {
                      n220 = Number To Boolean Array(number=u8 0) -> (Boolean array=w455:bool[])
                      n221 = local write "A_1"(w455) -> ()
                    }
                    frame 2 {
                      n222 = Number To Boolean Array(number=u8 0) -> (Boolean array=w457:bool[])
                      n223 = local write "A_2"(w457) -> ()
                    }
                    frame 3 {
                      n224 = Number To Boolean Array(number=u8 0) -> (Boolean array=w459:bool[])
                      n225 = local write "A_3"(w459) -> ()
                    }
                    frame 4 {
                      n226 = Number To Boolean Array(number=u8 0) -> (Boolean array=w461:bool[])
                      n227 = local write "A_4"(w461) -> ()
                    }
                    frame 5 {
                      n228 = Number To Boolean Array(number=u8 0) -> (Boolean array=w463:bool[])
                      n229 = local write "A_5"(w463) -> ()
                    }
                    frame 6 {
                      n230 = Number To Boolean Array(number=u8 0) -> (Boolean array=w465:bool[])
                      n231 = local write "A_6"(w465) -> ()
                    }
                    frame 7 {
                      n232 = Number To Boolean Array(number=u8 0) -> (Boolean array=w467:bool[])
                      n233 = local write "A_7"(w467) -> ()
                    }
                    frame 8 {
                      n234 = Number To Boolean Array(number=u8 0) -> (Boolean array=w469:bool[])
                      n235 = local write "A_8"(w469) -> ()
                    }
                    frame 9 {
                      n236 = Number To Boolean Array(number=u8 0) -> (Boolean array=w471:bool[])
                      n237 = local write "A_9"(w471) -> ()
                    }
                    frame 10 {
                      n238 = Number To Boolean Array(number=u8 0) -> (Boolean array=w473:bool[])
                      n239 = local write "A_10"(w473) -> ()
                    }
                    frame 11 {
                      n240 = Number To Boolean Array(number=u8 0) -> (Boolean array=w475:bool[])
                      n241 = local write "A_11"(w475) -> ()
                    }
                    frame 12 {
                      n242 = Number To Boolean Array(number=u8 0) -> (Boolean array=w477:bool[])
                      n243 = local write "A_12"(w477) -> ()
                    }
                    frame 13 {
                      n244 = Number To Boolean Array(number=u8 0) -> (Boolean array=w478:bool[])
                      n245 = local write "A_13"(w478) -> ()
                    }
                    frame 14 {
                      n246 = Number To Boolean Array(number=u8 0) -> (Boolean array=w481:bool[])
                      n247 = local write "A_14"(w481) -> ()
                    }
                    frame 15 {
                      n248 = Number To Boolean Array(number=u8 0) -> (Boolean array=w483:bool[])
                      n249 = local write "A_15"(w483) -> ()
                    }
                    frame 16 {
                      n250 = Number To Boolean Array(number=u8 0) -> (Boolean array=w485:bool[])
                      n251 = local write "A_16"(w485) -> ()
                    }
                  }
                }
                frame True {
                  # "Long cadena antes \nde ?"
                  # "Lee datos de puerto y desgloza Edif - Aula"
                  n252 = VISA Read(VISA resource name=w486, byte count=w496, error in (no error)=w497) -> (VISA resource name out=w495:refnum<visa-resource-name>, read buffer=w493:string, error out=w494:errorcluster)  [unwired: 1 out]
                  n253 = Search/Split String(string=w493, search string/char (-)="?", offset (0)=u8 0) -> (substring before match=w487:string)  [unwired: 2 out]
                  n254 = String Length(string=w487) -> (length=w489:i32)
                  n255 = Equal?(x=w489, y=4) -> (x = y?=w488:bool)
                  n256 = case shown="True" w488 {
                    tunnel: w487 -> [_ w499]
                    frame False {
                    }
                    frame True {
                      w498 = path "C:/BD_Monitor/LK__logger.udl" ("path")
                      # "Extrae 3er char\nservicios"
                      # "Extrae 1er char\nEdificio"
                      # "Segura long de cadena valida"
                      n257 = global write "Global_linker_path_logger.vi" "LK_logger"(w498) -> ()
                      n258 = String Subset(string=w499, offset (0)=u8 0, length (rest)=u8 1 ("length (rest)")) -> (substring=w504:string)
                      n259 = call-poly <vilib>:"DB Tools Open Connection.vi"("connection information"=w498) -> ("error out"=w503:errorcluster, "connection reference"=w502:T3)  [unwired: 7 in]
                      n260 = case shown="\"A\", Default" w504 {
                        tunnel: w499 -> [_ w514]
                        tunnel: w504 -> [_ w527]
                        tunnel: [w508 w525] -> w500
                        tunnel: [w507 w524] -> w501
                        tunnel: w503 -> [w507 w523]
                        tunnel: w502 -> [w508 w522]
                        frame "B" {
                        }
                        frame "A", Default {
                          # "4 char, \nde inactividad"
                          # "Extrae 2o char\nAula"
                          # "Detecta Edificio"
                          n261 = String Subset(string=w514, offset (0)=u8 2, length (rest)=u8 1 ("length (rest)")) -> (substring=w536:string)
                          n262 = local read "Numeric"() -> (w511:i32)
                          n263 = global read "contador_logger_global.vi" "log_count"() -> (w521:u64)
                          n264 = String Subset(string=w514, offset (0)=u8 1, length (rest)=u8 1 ("length (rest)")) -> (substring=w553:string)
                          n265 = Get Date/Time String(want seconds? (F)=TRUE) -> (date string=w546:string, time string=w547:string)  [unwired: 2 in]
                          n266 = Type Cast(type=u8 0 ("width (-)"), x=w536) -> (*(type *) &x=w541:u8)
                          n267 = Type Cast(type=u8 0 ("width (-)"), x=w553) -> (*(type *) &x=w551:u8)
                          n268 = Subtract(x=w541, y=u8 33) -> (x-y=w542:u8)
                          n269 = Equal?(x=w511, y=1) -> (x = y?=w512:bool)
                          n270 = Concatenate Strings(w546, "  " ("string"), w547) -> (w548:string)
                          n271 = Subtract(x=w551, y=u8 33) -> (x-y=w526:u8)
                          n272 = Increment(x=w521) -> (x+1=w516:u64)
                          n273 = Number To Boolean Array(number=w542) -> (Boolean array=w528:bool[])
                          n274 = call "subVi_extr_serv.vi"("Servicios_Edif"=w528) -> ("serv"=w549:string)
                          n275 = Bundle(w516, w548, "read buffer"=w527, w526, "serv"=w549) -> (w545:T4)  [unwired: 1 in]
                          n276 = case shown="True" w512 {
                            tunnel: w545 -> [_ w563]
                            tunnel: [w556 w562] -> w525
                            tunnel: [w557 w561] -> w524
                            tunnel: w523 -> [w557 w560]
                            tunnel: w522 -> [w556 w559]
                            frame False {
                            }
                            frame True {
                              n277 = call <vilib>:"DB Tools Insert Data.vi"("data"=w563, "error in (no error)"=w560, "table"="logs", "connection reference"=w559) -> ("error out"=w561:errorcluster, "connection reference out"=w562:T3)  [unwired: 6 in]
                            }
                          }
                          n278 = global write "contador_logger_global.vi" "log_count"(w516) -> ()
                          n279 = String Subset(string=w514, offset (0)=u8 3, length (rest)=u8 1 ("length (rest)")) -> (substring=w535:string)
                          n280 = Type Cast(type=u8 0 ("width (-)"), x=w535) -> (*(type *) &x=w534:u8)
                          n281 = Number To Decimal String(number=w516) -> (decimal integer string=w517:string)  [unwired: 1 in]
                          n282 = Subtract(x=w534, y=u8 33) -> (x-y=w529:u8)
                          n283 = case shown="1" w526 {
                            tunnel: w529 -> [_ w565 w570 w576 w582 w588 w594 w600 w606 w612 w618 w624 w630 w636 w642 w648 w654]
                            tunnel: w528 -> [_ w564 w571 w577 w583 w589 w595 w601 w607 w613 w619 w625 w631 w637 w643 w649 w655]
                            frame 0 {
                            }
                            frame 1 {
                              # "Detecta Aula"
                              n284 = case shown="1" w565 {
                                frame 0, Default {
                                n285 = property on="inc_1" class="Bool (strict)"("Blinking"=FALSE) -> ()  [unwired: 2 in, 2 out]
                                n286 = property on="inc_1" class="Bool (strict)"("Visible"=FALSE) -> ()  [unwired: 2 in, 2 out]
                                }
                                frame 1 {
                                n287 = property on="inc_1" class="Bool (strict)"("Blinking"=TRUE) -> ()  [unwired: 2 in, 2 out]
                                n288 = property on="inc_1" class="Bool (strict)"("Visible"=TRUE) -> ()  [unwired: 2 in, 2 out]
                                }
                              }
                              "A_1" <- w564
                            }
                            frame 2 {
                              n289 = case shown="0, Default" w570 {
                                frame 0, Default {
                                n290 = property on="inc_2" class="Bool (strict)"("Blinking"=FALSE) -> ()  [unwired: 2 in, 2 out]
                                n291 = property on="inc_2" class="Bool (strict)"("Visible"=FALSE) -> ()  [unwired: 2 in, 2 out]
                                }
                                frame 1 {
                                n292 = property on="inc_2" class="Bool (strict)"("Blinking"=TRUE) -> ()  [unwired: 2 in, 2 out]
                                n293 = property on="inc_2" class="Bool (strict)"("Visible"=TRUE) -> ()  [unwired: 2 in, 2 out]
                                }
                              }
                              "A_2" <- w571
                            }
                            frame 3 {
                              n294 = case shown="0, Default" w576 {
                                frame 0, Default {
                                n295 = property on="inc_3" class="Bool (strict)"("Blinking"=FALSE) -> ()  [unwired: 2 in, 2 out]
                                n296 = property on="inc_3" class="Bool (strict)"("Visible"=FALSE) -> ()  [unwired: 2 in, 2 out]
                                }
                                frame 1 {
                                n297 = property on="inc_3" class="Bool (strict)"("Blinking"=TRUE) -> ()  [unwired: 2 in, 2 out]
                                n298 = property on="inc_3" class="Bool (strict)"("Visible"=TRUE) -> ()  [unwired: 2 in, 2 out]
                                }
                              }
                              "A_3" <- w577
                            }
                            frame 4 {
                              n299 = case shown="0, Default" w582 {
                                frame 0, Default {
                                n300 = property on="inc_4" class="Bool (strict)"("Blinking"=FALSE) -> ()  [unwired: 2 in, 2 out]
                                n301 = property on="inc_4" class="Bool (strict)"("Visible"=FALSE) -> ()  [unwired: 2 in, 2 out]
                                }
                                frame 1 {
                                n302 = property on="inc_4" class="Bool (strict)"("Blinking"=TRUE) -> ()  [unwired: 2 in, 2 out]
                                n303 = property on="inc_4" class="Bool (strict)"("Visible"=TRUE) -> ()  [unwired: 2 in, 2 out]
                                }
                              }
                              "A_4" <- w583
                            }
                            frame 5 {
                              n304 = case shown="0, Default" w588 {
                                frame 0, Default {
                                n305 = property on="inc_5" class="Bool (strict)"("Blinking"=FALSE) -> ()  [unwired: 2 in, 2 out]
                                n306 = property on="inc_5" class="Bool (strict)"("Visible"=FALSE) -> ()  [unwired: 2 in, 2 out]
                                }
                                frame 1 {
                                n307 = property on="inc_5" class="Bool (strict)"("Blinking"=TRUE) -> ()  [unwired: 2 in, 2 out]
                                n308 = property on="inc_5" class="Bool (strict)"("Visible"=TRUE) -> ()  [unwired: 2 in, 2 out]
                                }
                              }
                              "A_5" <- w589
                            }
                            frame 6 {
                              n309 = case shown="0, Default" w594 {
                                frame 0, Default {
                                n310 = property on="inc_6" class="Bool (strict)"("Blinking"=FALSE) -> ()  [unwired: 2 in, 2 out]
                                n311 = property on="inc_6" class="Bool (strict)"("Visible"=FALSE) -> ()  [unwired: 2 in, 2 out]
                                }
                                frame 1 {
                                n312 = property on="inc_6" class="Bool (strict)"("Blinking"=TRUE) -> ()  [unwired: 2 in, 2 out]
                                n313 = property on="inc_6" class="Bool (strict)"("Visible"=TRUE) -> ()  [unwired: 2 in, 2 out]
                                }
                              }
                              "A_6" <- w595
                            }
                            frame 7 {
                              n314 = case shown="0, Default" w600 {
                                frame 0, Default {
                                n315 = property on="inc_7" class="Bool (strict)"("Blinking"=FALSE) -> ()  [unwired: 2 in, 2 out]
                                n316 = property on="inc_7" class="Bool (strict)"("Visible"=FALSE) -> ()  [unwired: 2 in, 2 out]
                                }
                                frame 1 {
                                n317 = property on="inc_7" class="Bool (strict)"("Blinking"=TRUE) -> ()  [unwired: 2 in, 2 out]
                                n318 = property on="inc_7" class="Bool (strict)"("Visible"=TRUE) -> ()  [unwired: 2 in, 2 out]
                                }
                              }
                              "A_7" <- w601
                            }
                            frame 8 {
                              n319 = case shown="0, Default" w606 {
                                frame 0, Default {
                                n320 = property on="inc_8" class="Bool (strict)"("Blinking"=FALSE) -> ()  [unwired: 2 in, 2 out]
                                n321 = property on="inc_8" class="Bool (strict)"("Visible"=FALSE) -> ()  [unwired: 2 in, 2 out]
                                }
                                frame 1 {
                                n322 = property on="inc_8" class="Bool (strict)"("Blinking"=TRUE) -> ()  [unwired: 2 in, 2 out]
                                n323 = property on="inc_8" class="Bool (strict)"("Visible"=TRUE) -> ()  [unwired: 2 in, 2 out]
                                }
                              }
                              "A_8" <- w607
                            }
                            frame 9 {
                              n324 = case shown="0, Default" w612 {
                                frame 0, Default {
                                n325 = property on="inc_9" class="Bool (strict)"("Blinking"=FALSE) -> ()  [unwired: 2 in, 2 out]
                                n326 = property on="inc_9" class="Bool (strict)"("Visible"=FALSE) -> ()  [unwired: 2 in, 2 out]
                                }
                                frame 1 {
                                n327 = property on="inc_9" class="Bool (strict)"("Blinking"=TRUE) -> ()  [unwired: 2 in, 2 out]
                                n328 = property on="inc_9" class="Bool (strict)"("Visible"=TRUE) -> ()  [unwired: 2 in, 2 out]
                                }
                              }
                              "A_9" <- w613
                            }
                            frame 10 {
                              n329 = case shown="0, Default" w618 {
                                frame 0, Default {
                                n330 = property on="inc_10" class="Bool (strict)"("Blinking"=FALSE) -> ()  [unwired: 2 in, 2 out]
                                n331 = property on="inc_10" class="Bool (strict)"("Visible"=FALSE) -> ()  [unwired: 2 in, 2 out]
                                }
                                frame 1 {
                                n332 = property on="inc_10" class="Bool (strict)"("Blinking"=TRUE) -> ()  [unwired: 2 in, 2 out]
                                n333 = property on="inc_10" class="Bool (strict)"("Visible"=TRUE) -> ()  [unwired: 2 in, 2 out]
                                }
                              }
                              "A_10" <- w619
                            }
                            frame 11 {
                              n334 = case shown="0, Default" w624 {
                                frame 0, Default {
                                n335 = property on="inc_11" class="Bool (strict)"("Blinking"=FALSE) -> ()  [unwired: 2 in, 2 out]
                                n336 = property on="inc_11" class="Bool (strict)"("Visible"=FALSE) -> ()  [unwired: 2 in, 2 out]
                                }
                                frame 1 {
                                n337 = property on="inc_11" class="Bool (strict)"("Blinking"=TRUE) -> ()  [unwired: 2 in, 2 out]
                                n338 = property on="inc_11" class="Bool (strict)"("Visible"=TRUE) -> ()  [unwired: 2 in, 2 out]
                                }
                              }
                              "A_11" <- w625
                            }
                            frame 12 {
                              n339 = case shown="0, Default" w630 {
                                frame 0, Default {
                                n340 = property on="inc_12" class="Bool (strict)"("Blinking"=FALSE) -> ()  [unwired: 2 in, 2 out]
                                n341 = property on="inc_12" class="Bool (strict)"("Visible"=FALSE) -> ()  [unwired: 2 in, 2 out]
                                }
                                frame 1 {
                                n342 = property on="inc_12" class="Bool (strict)"("Blinking"=TRUE) -> ()  [unwired: 2 in, 2 out]
                                n343 = property on="inc_12" class="Bool (strict)"("Visible"=TRUE) -> ()  [unwired: 2 in, 2 out]
                                }
                              }
                              "A_12" <- w631
                            }
                            frame 13 {
                              n344 = case shown="1" w636 {
                                frame 0, Default {
                                n345 = property on="inc_13" class="Bool (strict)"("Blinking"=FALSE) -> ()  [unwired: 2 in, 2 out]
                                n346 = property on="inc_13" class="Bool (strict)"("Visible"=FALSE) -> ()  [unwired: 2 in, 2 out]
                                }
                                frame 1 {
                                n347 = property on="inc_13" class="Bool (strict)"("Blinking"=TRUE) -> ()  [unwired: 2 in, 2 out]
                                n348 = property on="inc_13" class="Bool (strict)"("Visible"=TRUE) -> ()  [unwired: 2 in, 2 out]
                                }
                              }
                              "A_13" <- w637
                            }
                            frame 14 {
                              n349 = case shown="0, Default" w642 {
                                frame 0, Default {
                                n350 = property on="inc_14" class="Bool (strict)"("Blinking"=FALSE) -> ()  [unwired: 2 in, 2 out]
                                n351 = property on="inc_14" class="Bool (strict)"("Visible"=FALSE) -> ()  [unwired: 2 in, 2 out]
                                }
                                frame 1 {
                                n352 = property on="inc_14" class="Bool (strict)"("Blinking"=TRUE) -> ()  [unwired: 2 in, 2 out]
                                n353 = property on="inc_14" class="Bool (strict)"("Visible"=TRUE) -> ()  [unwired: 2 in, 2 out]
                                }
                              }
                              "A_14" <- w643
                            }
                            frame 15, Default {
                              n354 = case shown="0, Default" w648 {
                                frame 0, Default {
                                n355 = property on="inc_15" class="Bool (strict)"("Blinking"=FALSE) -> ()  [unwired: 2 in, 2 out]
                                n356 = property on="inc_15" class="Bool (strict)"("Visible"=FALSE) -> ()  [unwired: 2 in, 2 out]
                                }
                                frame 1 {
                                n357 = property on="inc_15" class="Bool (strict)"("Blinking"=TRUE) -> ()  [unwired: 2 in, 2 out]
                                n358 = property on="inc_15" class="Bool (strict)"("Visible"=TRUE) -> ()  [unwired: 2 in, 2 out]
                                }
                              }
                              "A_15" <- w649
                            }
                            frame 16 {
                              n359 = case shown="0, Default" w654 {
                                frame 0, Default {
                                n360 = property on="inc_16" class="Bool (strict)"("Blinking"=FALSE) -> ()  [unwired: 2 in, 2 out]
                                n361 = property on="inc_16" class="Bool (strict)"("Visible"=FALSE) -> ()  [unwired: 2 in, 2 out]
                                }
                                frame 1 {
                                n362 = property on="inc_16" class="Bool (strict)"("Blinking"=TRUE) -> ()  [unwired: 2 in, 2 out]
                                n363 = property on="inc_16" class="Bool (strict)"("Visible"=TRUE) -> ()  [unwired: 2 in, 2 out]
                                }
                              }
                              "A_16" <- w655
                            }
                          }
                          n364 = Open/Create/Replace File(file path (use dialog)=path "C:/BD_Monitor/contador_logg.txt" ("path"), operation (0:open)=T1."replace or create") -> (refnum out=w513:refnum<file>, error out=w520:errorcluster)  [unwired: 4 in, 1 out]
                          n365 = Write to Text File(file (use dialog)=w513, text=w517, error in=w520) -> (refnum out=w515:refnum<file>, error out=w519:errorcluster)  [unwired: 1 in, 1 out]
                          n366 = Close File(refnum=w515, error in=w519) -> ()  [unwired: 2 out]
                        }
                      }
                      n367 = call <vilib>:"DB Tools Close Connection.vi"("error in (no error)"=w501, "connection reference"=w500) -> ()  [unwired: 5 in, 1 out]
                    }
                  }
                }
              }
              "Numeric" <- w427
            }
          }
        }
      }
      frame False {
      }
    }
  }
  n368 = while {
    stop <- "Stop Button" stop-if-true
    # "hora de arranque\nde ejecutor"
    # "Ciclo  para Abrir Sub - programas --> programador de tareas, & ejecucion manual; goto tareas programadas"
    n369 = Wait Until Next ms Multiple(millisecond multiple=u32 100) -> ()  [unwired: 1 out]
    n370 = Get Date/Time In Seconds() -> (seconds since 1Jan1904=w675:timestamp)
    n371 = Or(x="Programar Tareas", y="Programar Tareas2") -> (x .or. y?=w678:bool)
    n372 = case shown="True" w678 {
      frame False {
      }
      frame True {
        n373 = global write "GlobalFag.vi" "Boolean"(TRUE ("Boolean")) -> ()
        n374 = Current VI's Path() -> (path=w688:path)
        n375 = Build Path(base path=w688, name or relative path=path "../Form_progr_tareas.vi" ("path")) -> (appended path=w686:path)
        n376 = Open VI Reference(vi path=w686) -> (vi reference=w700:refnum<vi>, error out=w699:errorcluster)  [unwired: 5 in]
        n377 = local write "Programar Tareas"(FALSE ("OK Button")) -> ()
        n378 = invoke class="VI" method="FP.Open"(reference=w700, error in=w699, "Activate"=FALSE ("Activate?"), "State"=T5."Standard") -> (reference out=w695:refnum<vi>, error out=w694:errorcluster)  [unwired: 1 in, 3 out]
        n379 = invoke class="VI" method="FP.Center"(reference=w695, error in=w694) -> (reference out=w689:refnum<vi>, error out=w693:errorcluster)  [unwired: 1 in, 1 out]
        n380 = invoke class="VI" method="Run VI"(reference=w689, error in=w693) -> (reference out=w697:refnum<vi>, error out=w696:errorcluster)  [unwired: 3 in, 3 out]
        n381 = Close Reference(reference=w697, error in (no error)=w696) -> ()  [unwired: 1 out]
      }
    }
    n382 = case shown="True" "Manual Aula / Edificio" {
      frame False {
      }
      frame True {
        n383 = global write "GlobalFag.vi" "Boolean"(FALSE ("Boolean")) -> ()
        n384 = Current VI's Path() -> (path=w703:path)
        n385 = Build Path(base path=w703, name or relative path=path "../Ejecutor_manual.vi" ("path")) -> (appended path=w701:path)
        n386 = Open VI Reference(vi path=w701) -> (vi reference=w715:refnum<vi>, error out=w714:errorcluster)  [unwired: 5 in]
        n387 = local write "Manual Aula / Edificio"(FALSE ("OK Button")) -> ()
        n388 = invoke class="VI" method="FP.Open"(reference=w715, error in=w714, "Activate"=FALSE ("Activate?"), "State"=T5."Standard") -> (reference out=w710:refnum<vi>, error out=w709:errorcluster)  [unwired: 1 in, 3 out]
        n389 = invoke class="VI" method="FP.Center"(reference=w710, error in=w709) -> (reference out=w707:refnum<vi>, error out=w708:errorcluster)  [unwired: 1 in, 1 out]
        n390 = invoke class="VI" method="Run VI"(reference=w707, error in=w708) -> (reference out=w712:refnum<vi>, error out=w711:errorcluster)  [unwired: 3 in, 3 out]
        n391 = Close Reference(reference=w712, error in (no error)=w711) -> ()  [unwired: 1 out]
      }
    }
    n392 = case shown="True" "Ejecutor de Tareas" {
      frame False {
      }
      frame True {
        n393 = property on="Pane" class="Pane"("Origin"=T2 {"Horizontal"=1833, "Vertical"=-110}) -> ()  [unwired: 2 in, 2 out]
      }
    }
    n394 = Get Date/Time String(seconds (now)=w675, want seconds? (F)=TRUE) -> (time string=w672:string)  [unwired: 1 in, 1 out]
    n395 = Scan From String(format string="%<%I:%M:%S %p>T", input string="01:00:00 a. m.") -> (output 1=w665:timestamp)  [unwired: 3 in, 3 out]
    n396 = Scan From String(format string="%<%I:%M:%S %p>T", input string=w672) -> (output 1=w664:timestamp)  [unwired: 3 in, 3 out]
    n397 = Add(x=w665, y=u16 900) -> (x+y=w666:timestamp)
    n398 = Greater Or Equal?(x=w664, y=w665) -> (x >= y?=w668:bool)
    n399 = Less Or Equal?(x=w664, y=w666) -> (x <= y?=w667:bool)
    n400 = And(x=w668, y=w667) -> (x .and. y?=w663:bool)
    n401 = case shown="True" w663 {
      frame False {
      }
      frame True {
        w683 = TRUE ("act_aula")
        n402 = global write "global_act_eje_edif.vi" "act_prog_edif"(w683) -> ()
        n403 = global write "global_act_eje_aula.vi" "act_aula"(w683) -> ()
      }
    }
    n404 = case shown="True" "Home Button" {
      frame False {
      }
      frame True {
        n405 = property on="Pane" class="Pane"("Origin"=T2 {"Horizontal"=-53, "Vertical"=-110}) -> ()  [unwired: 2 in, 2 out]
      }
    }
  }
  n406 = call <vilib>:"DB Tools Close Connection.vi"("error in (no error)"=w15, "connection reference"=w14) -> ()  [unwired: 5 in, 1 out]
  n407 = call <vilib>:"DB Tools Close Connection.vi"("error in (no error)"=w21, "connection reference"=w22) -> ()  [unwired: 5 in, 1 out]
  n408 = VISA Close(VISA resource name=w39, error in (no error)=w37) -> ()  [unwired: 1 out]
  "inc_14" <- w28
  "inc_15" <- w28
  "inc_16" <- w28
  "inc_12" <- w28
  "inc_11" <- w28
  "inc_10" <- w28
  "inc_9" <- w28
  "inc_8" <- w28
  "inc_7" <- w28
  "inc_6" <- w28
  "inc_13" <- w28
  "inc_2" <- w28
  "inc_4" <- w28
  "inc_3" <- w28
  "inc_5" <- w28
  "inc_1" <- w28
